vi "Angle to Unit Circle.vi"(11 "Actual Angle":dbl) -> (3 "Unit Circle Angle":dbl)   [LabVIEW 2016]
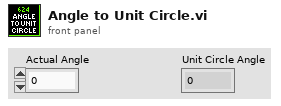
[diagram p1: front panel]
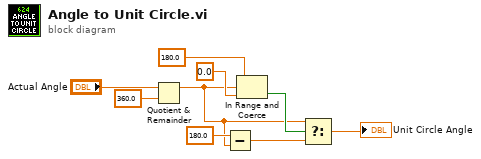
[diagram p0: block diagram]
diagram:
  n1 = Quotient & Remainder(x="Actual Angle", y=360.0) -> (x-y*floor(x/y)=w2:dbl)  [unwired: 1 out]
  n2 = Subtract(x=180.0 ("y"), y=w2) -> (x-y=w1:dbl)
  n3 = In Range and Coerce(upper limit=180.0, x=w2, lower limit=0.0) -> (In Range?=w5:bool)  [unwired: 1 out]
  n4 = Select(t=w2, s=w5, f=w1) -> (s? t:f=→"Unit Circle Angle":dbl)
